vi "sendInt.vi"(0 "VISA resource name":refnum<visa-resource-name>, 5 "number":u16(slide) max=999 step=1 scale=0.0..999.0, 7 "letter":string, 9 "sender":bool, 11 "error in (no error)":errorcluster) -> (4 "VISA resource name out":refnum<visa-resource-name>, 15 "error out":errorcluster)   [LabVIEW 2013]
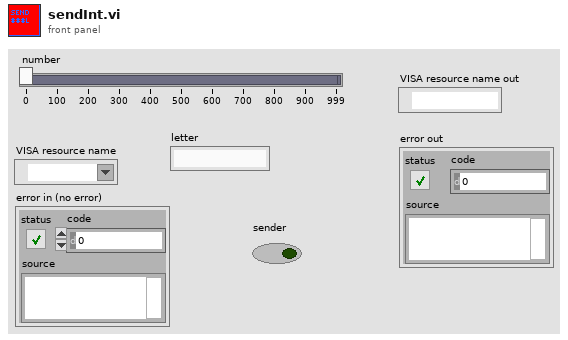
[diagram p1: front panel]
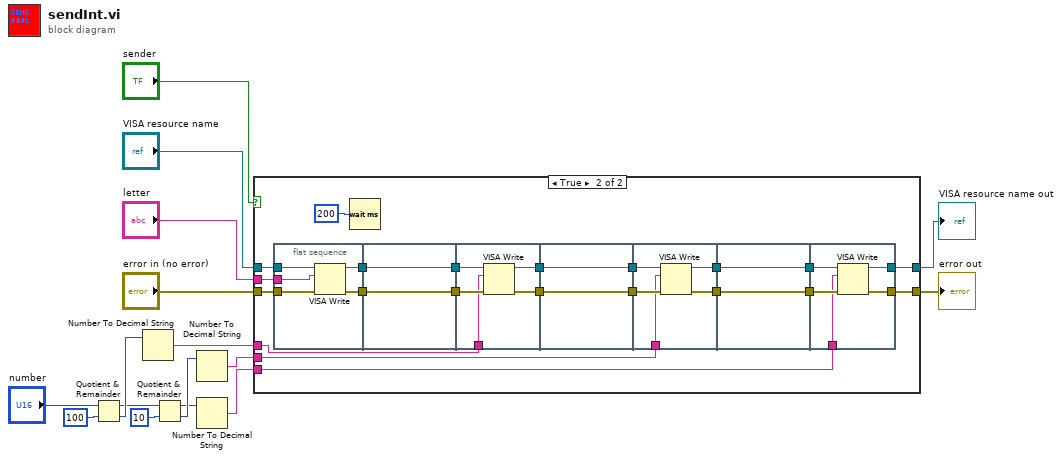
[diagram p0: block diagram]
diagram:
  n1 = Quotient & Remainder(x="number", y=u16 100) -> (x-y*floor(x/y)=w13:u16, floor(x/y)=w14:u16)
  n2 = Number To Decimal String(number=w14) -> (decimal integer string=w9:string)  [unwired: 1 in]
  n3 = Quotient & Remainder(x=w13, y=u16 10) -> (x-y*floor(x/y)=w10:u16, floor(x/y)=w11:u16)
  n4 = Number To Decimal String(number=w11) -> (decimal integer string=w8:string)  [unwired: 1 in]
  n5 = Number To Decimal String(number=w10) -> (decimal integer string=w1:string)  [unwired: 1 in]
  n6 = case shown="True" "sender" {
    tunnel: w9 -> [_ w23]
    tunnel: w8 -> [_ w22]
    tunnel: w1 -> [_ w21]
    tunnel: "letter" -> [_ w36]
    tunnel: "VISA resource name" -> [w18 w38]
    tunnel: "error in (no error)" -> [w17 w37]
    tunnel: [w18 w20] -> w3
    tunnel: [w17 w19] -> w2
    frame False {
    }
    frame True {
      n7 = flat-sequence {
        tunnel: w38 -> [w44]
        tunnel: w37 -> [w43]
        tunnel: w36 -> [w42]
        tunnel: [w41] -> w34
        tunnel: [w40] -> w28
        tunnel: [w46] -> w35
        tunnel: w34 -> [w46]
        tunnel: [w45] -> w29
        tunnel: w28 -> [w45]
        tunnel: w35 -> [w51]
        tunnel: [w50] -> w32
        tunnel: w29 -> [w49]
        tunnel: [w48] -> w26
        tunnel: w23 -> [w47]
        tunnel: [w53] -> w33
        tunnel: w32 -> [w53]
        tunnel: [w52] -> w27
        tunnel: w26 -> [w52]
        tunnel: w33 -> [w58]
        tunnel: [w57] -> w30
        tunnel: w27 -> [w56]
        tunnel: [w55] -> w24
        tunnel: w22 -> [w54]
        tunnel: [w60] -> w31
        tunnel: w30 -> [w60]
        tunnel: [w59] -> w25
        tunnel: w24 -> [w59]
        tunnel: w31 -> [w65]
        tunnel: w25 -> [w64]
        tunnel: w21 -> [w63]
        tunnel: [w62] -> w20
        tunnel: [w61] -> w19
        frame #0 {
          n8 = VISA Write(VISA resource name=w44, write buffer=w42, error in (no error)=w43) -> (VISA resource name out=w41:refnum<visa-resource-name>, error out=w40:errorcluster)  [unwired: 1 out]
        }
        frame #1 {
        }
        frame #2 {
          n9 = VISA Write(VISA resource name=w51, write buffer=w47, error in (no error)=w49) -> (VISA resource name out=w50:refnum<visa-resource-name>, error out=w48:errorcluster)  [unwired: 1 out]
        }
        frame #3 {
        }
        frame #4 {
          n10 = VISA Write(VISA resource name=w58, write buffer=w54, error in (no error)=w56) -> (VISA resource name out=w57:refnum<visa-resource-name>, error out=w55:errorcluster)  [unwired: 1 out]
        }
        frame #5 {
        }
        frame #6 {
          n11 = VISA Write(VISA resource name=w65, write buffer=w63, error in (no error)=w64) -> (VISA resource name out=w62:refnum<visa-resource-name>, error out=w61:errorcluster)  [unwired: 1 out]
        }
      }
      n12 = Wait (ms)(milliseconds to wait=u32 200) -> ()  [unwired: 1 out]
    }
  }
  "VISA resource name out" <- w3
  "error out" <- w2
